vi "Init_Sys.vi"(9 "Password":string="admin", 10 "Username":string="admin", 11 "IP Address":string="192.168.0.1") -> (0 "error out":errorcluster, 2 "handle":i32, 3 "crate_map":string[][](table))   [LabVIEW 2018]
uses:
  <instrlib>/CAENHVWrapper/CAENHVWrapper.lvlib
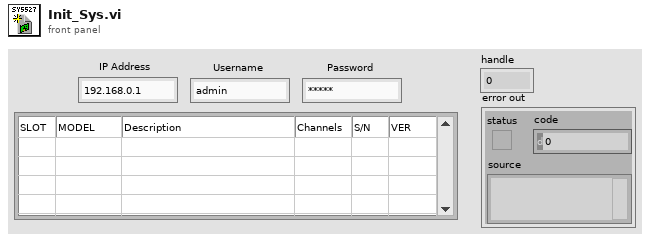
[diagram p1: front panel]
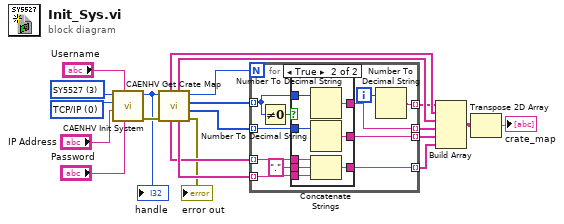
[diagram p0: block diagram]
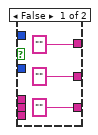
[diagram p2: hidden frame]
diagram:
  w17 = u32 3 items=["SY1527", "SY2527", "SY4527", "SY5527", "N568", "V65XX", "N1470", "V8100"] ("system")
  w18 = 0 items=["TCP/IP"=0, "HS CAENET"=2, "USB 2.0"=3, "CONET Optical Link"=4, "USB VCP"=5] ("LinkType")
  n1 = call <instrlib>:"CAENHV Init System.vi"("Passwd"="Password", "UserName"="Username", "Arg"="IP Address", "LinkType"=w18, "system"=w17) -> ("error out"=w5:errorcluster, "handle"=w1:i32)  [unwired: 5 in]
  "handle" <- w1
  n2 = call <instrlib>:"CAENHV Get Crate Map.vi"("error in (no error)"=w5, "handle"=w1) -> ("error out"=→"error out":errorcluster, "SerNumList"=w9:i16[], "NrofChList"=w13:i16[], "NrOfSlot"=w4:u16, "FmwRelMinList"=w7:string[], "DescriptionList"=w15:string[], "FmwRelMaxList"=w6:string[], "ModelList"=w16:string[])  [unwired: 2 in]
  n3 = for {
    N: w4 -> [_]
    tunnel: [w23] -> w14 mode=indexing
    tunnel: w13 -> [w25] mode=indexing
    tunnel: [w32] -> w12 mode=indexing
    tunnel: w9 -> [w31] mode=indexing
    tunnel: [w30] -> w8 mode=indexing
    tunnel: w7 -> [w27] mode=indexing
    tunnel: w6 -> [w29] mode=indexing
    tunnel: [w28] -> w3 mode=indexing
    i -> [w22]
    n4 = Not Equal To 0?(x=w25) -> (x != 0?=w24:bool)
    n5 = case shown="True" w24 {
      tunnel: ["" w43] -> w32
      tunnel: w31 -> [_ w42]
      tunnel: ["" w41] -> w30
      tunnel: w29 -> [_ w40]
      tunnel: ["" w39] -> w28
      tunnel: w27 -> [_ w38]
      tunnel: "." ("string") -> [_ w37]
      tunnel: w25 -> [_ w36]
      frame False {
      }
      frame True {
        n6 = Number To Decimal String(number=w36) -> (decimal integer string=w43:string)  [unwired: 1 in]
        n7 = Number To Decimal String(number=w42) -> (decimal integer string=w41:string)  [unwired: 1 in]
        n8 = Concatenate Strings(w40, w37, w38) -> (w39:string)
      }
    }
    n9 = Number To Decimal String(number=w22) -> (decimal integer string=w23:string)  [unwired: 1 in]
  }
  n10 = Build Array(w14, w16, w15, w12, w8, w3) -> (w11:string[][])
  n11 = Transpose 2D Array(2D array=w11) -> (transposed array=→"crate_map":string[][])
